vi "Init.vi"(8 "error in (no error)":errorcluster) -> (0 "error out":errorcluster, 3 "TelemetryService out":refnum<class "TelemetryService.lvclass">)   [LabVIEW 2020, in "Vecto.lvlib" / "TelemetryService.lvclass"]
uses:
  TelemetryService.lvclass
  TelemetryService.lvclass/TelemetryService.ctl
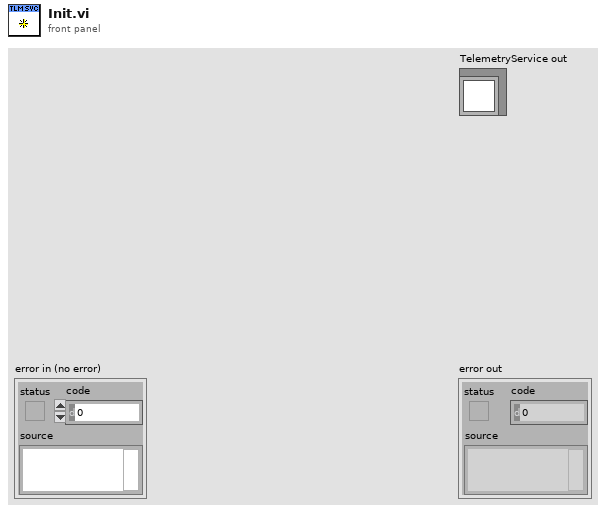
[diagram p1: front panel]
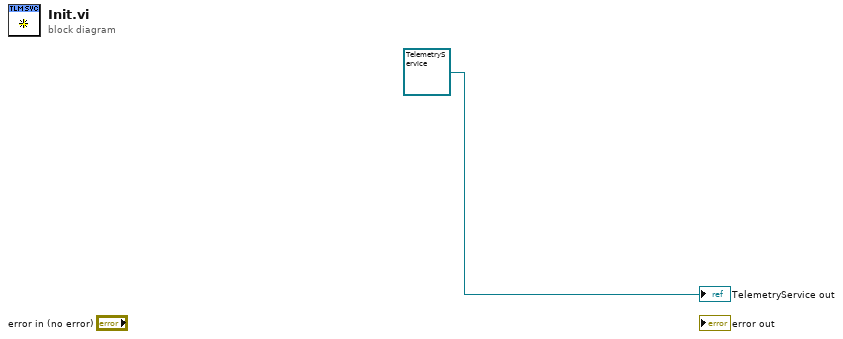
[diagram p0: block diagram]
diagram:
  "TelemetryService out" <- refnum<class "TelemetryService.lvclass"> refnum ("TelemetryService in")
